vi "Write Registry Value String.vi"(8 "error in (no error)":errorcluster, 9 "Value":string, 10 "Key":string, 11 "Path":string) -> (0 "error out":errorcluster, 1 "Value out":string, 2 "Key out":string, 3 "Path out":string, 5 "function return":bool)   [LabVIEW 2017, in "LumencorDLLDbg64.lvlib"]
doc: "This function Writes (overwrites) The Light Engine Color map to the registry.\nOnly use this function if instructed to by Lumencor.\n\n\n\nextern \"C\" LUMENCORDLL2B_API bool WriteRegistryValueString(LPSTR Path, LPSTR Key, LPSTR Value);"
uses:
  LumencorDLLDbg64.lvlib
  LumencorDLLDbg64.dll
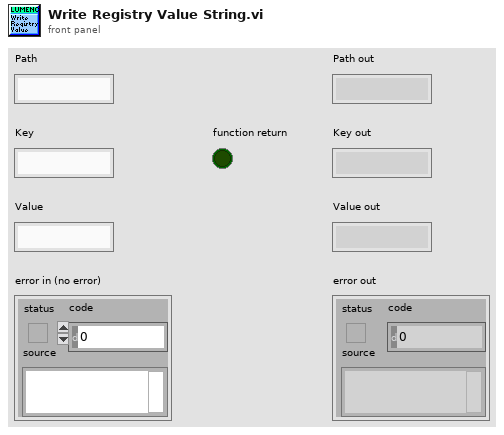
[diagram p1: front panel]
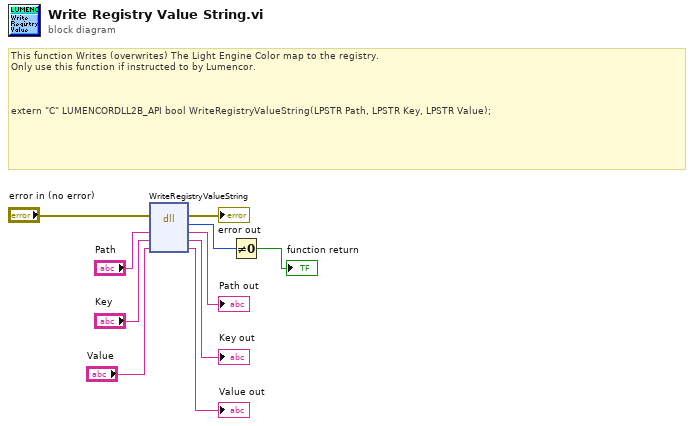
[diagram p0: block diagram]
diagram:
  # "This function Writes (overwrites) The Light Engine Color map to the registry.\nOnly use this function if instructed to by Lumencor.\n\n\n\nextern \"C\" LUMENCORDLL2B_API bool WriteRegistryValueString(LPSTR Path, LPSTR Key, LPSTR Value);"
  n1 = dll-call lib="Q:/GIT -- Lumencor DLL4/LabVIEW Library (64bit)/LumencorDLLDbg64.*" fn="WriteRegistryValueString"(error in="error in (no error)", "Path"="Path", "Key"="Key", "Value"="Value") -> (error out=→"error out":errorcluster, w9:u8, "Path"=→"Path out":string, "Key"=→"Key out":string, "Value"=→"Value out":string)  [unwired: 2 in, 1 out]
  n2 = Not Equal To 0?(x=w9) -> (x != 0?=→"function return":bool)
